vi "kalibrace.vi"() -> ()   [LabVIEW 2024]
uses:
  <vilib>/Analysis/baseanly.llb/Mean (DBL).vi
  EFmeter.lvlib
  <vilib>/Analysis/NI_AALBase.lvlib
  <vilib>/Analysis/NI_AALPro.lvlib
panel:
  out "Polynomial Coefficients":dbl[](array[numeric])
  out "Best Polynomial Fit":dbl[](array[numeric])
  in  "vyh\nVyhodnotit":bool
  in  "Další":bool caption="OK Button"
  in  "Reálná hodnota vstupní veličiny":dbl
  in  "Clear":bool
  in  "Uložit data":bool
  in  "file path (use dialog)":path
  in  "Vzorku na krokù":u16 max=100 step=1
  in  "Prumerovani":bool
  out "error out 2":errorcluster
  in  "VISA resource name 2":refnum<visa-resource-name>
  out "R_out":dbl
  out "XY Graph 2":cluster{"X":dbl[], "Y":dbl[]}[](graph)
  in  "stop":bool
  in  "Start":bool
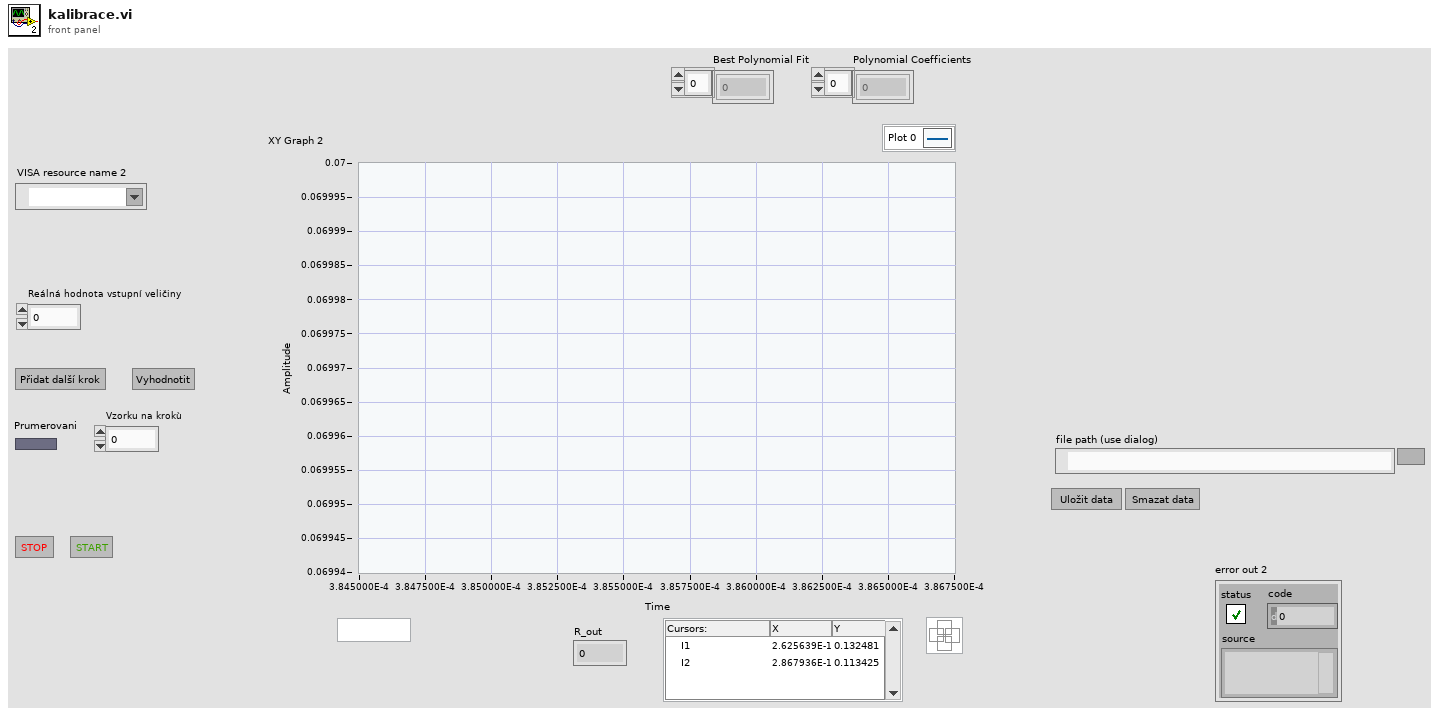
[diagram p1: front panel]
types:
  T1 = enum16{"init", "wait", "graph", "meas", "change_load", "init_measurment", "save", "clear"}
  T2 = typedef "LVCursorListTypeDef.ctl" = cluster{"Name":string, "Color":u32, "Style":u8, "Point Style":u8, "Name Visible":bool, "Allow Drag":bool, "Cursor Mode":u32, "Plot":i32, "Index":i32, "Position":cluster{"X":dbl, "Y":dbl}, "X Scale":u32, "Y Scale":u32, "Watch Plots":i32[], "Watch All Plots":bool, "Plot Area":i32, "Label Offset":cluster{"X":dbl, "Y":dbl}}[]
  T3 = cluster{"Name":string, "Color":u32, "Style":u8, "Point Style":u8, "Name Visible":bool, "Allow Drag":bool, "Cursor Mode":u32, "Plot":i32, "Index":i32, "Position":cluster{"X":dbl, "Y":dbl}, "X Scale":u32, "Y Scale":u32, "Watch Plots":i32[], "Watch All Plots":bool, "Plot Area":i32, "Label Offset":cluster{"X":dbl, "Y":dbl}}
  T4 = enum16{"open", "replace", "create", "open or create", "replace or create", "replace or create with confirmation"}
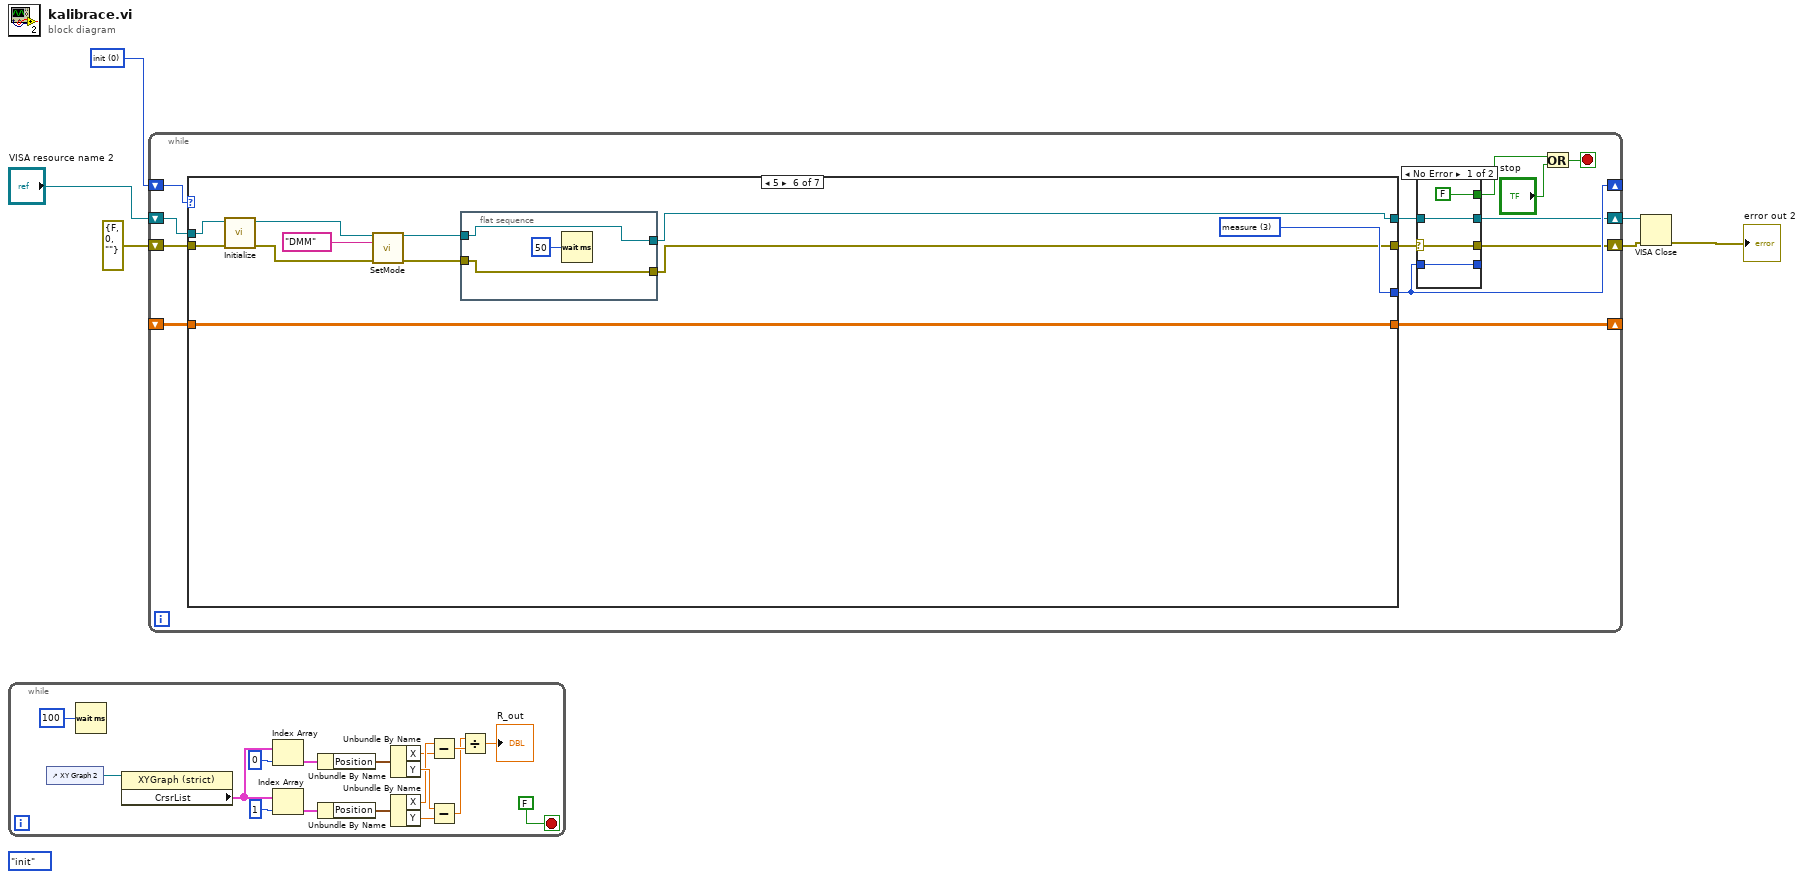
[diagram p0: block diagram]
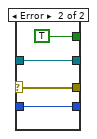
[diagram p2: hidden frame]
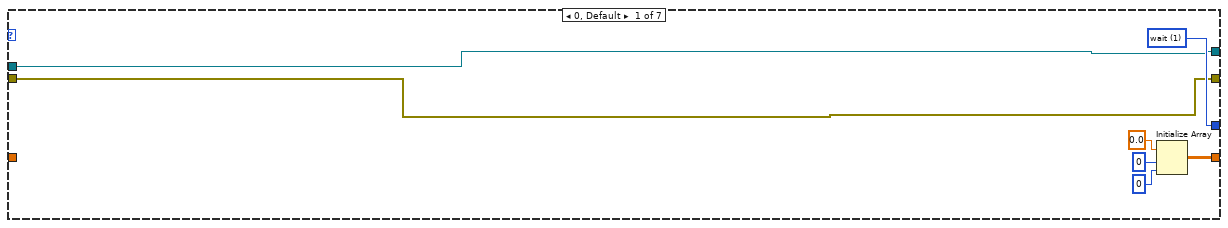
[diagram p3: hidden frame]
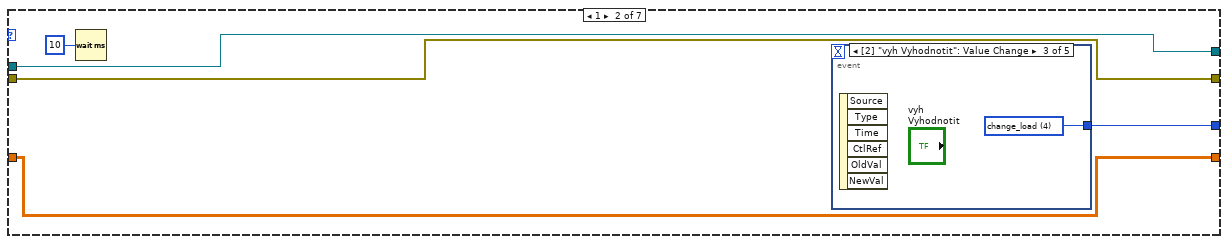
[diagram p4: hidden frame]
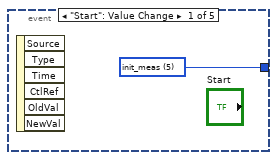
[diagram p5: hidden frame]
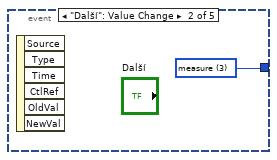
[diagram p6: hidden frame]
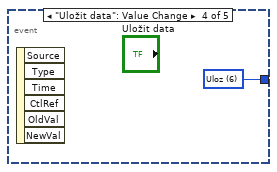
[diagram p7: hidden frame]
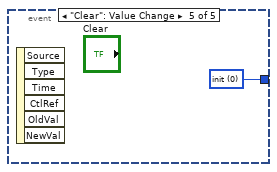
[diagram p8: hidden frame]
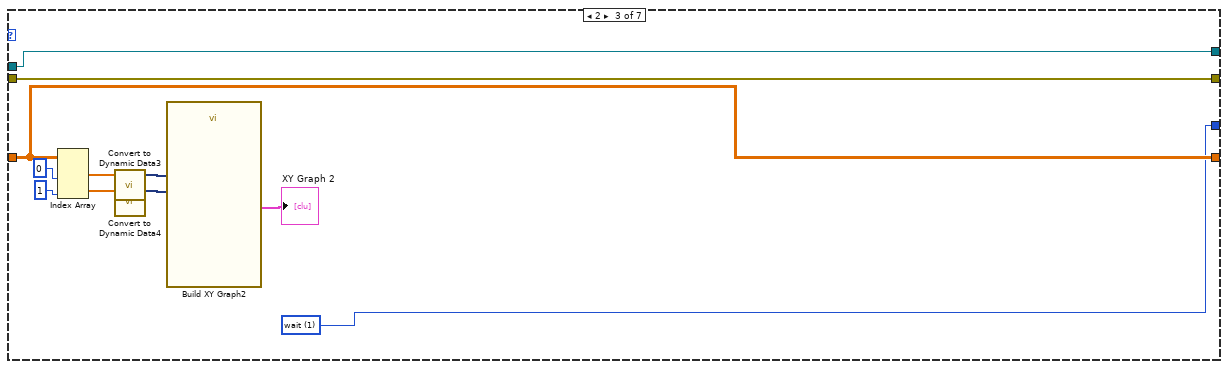
[diagram p9: hidden frame]
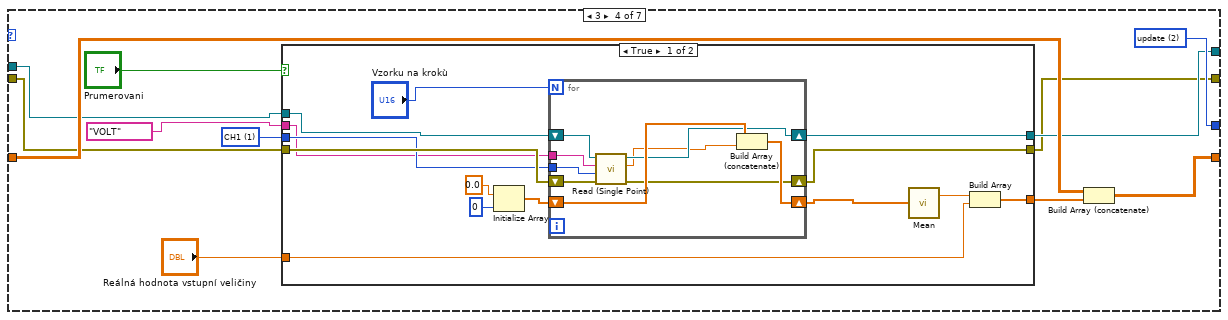
[diagram p10: hidden frame]
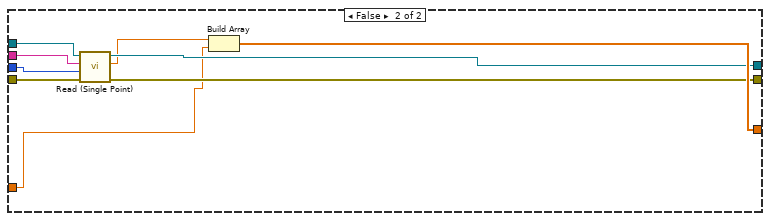
[diagram p11: hidden frame]
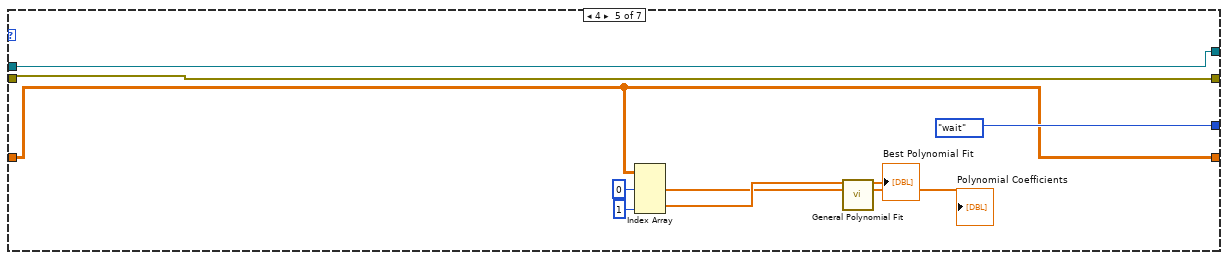
[diagram p12: hidden frame]
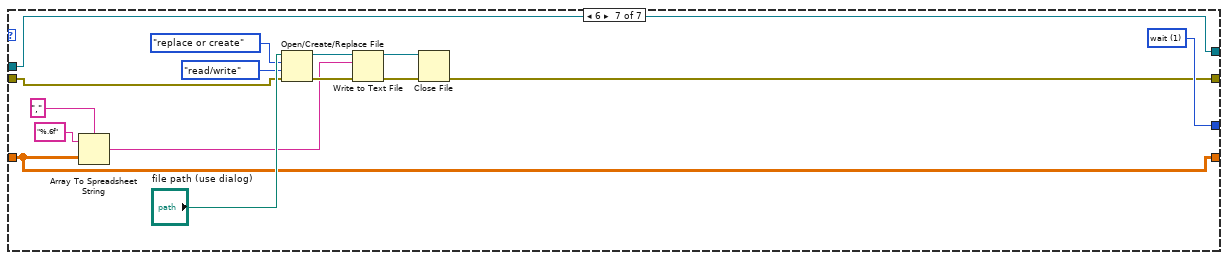
[diagram p13: hidden frame]
diagram:
  (unwired) T1."init"
  w6 = u16 0 items=["init", "wait", "update", "measure", "change_load", "init_meas", "Uloz", "clear"]
  n1 = while {
    stop <- FALSE stop-if-true
    n2 = control-ref of="XY Graph 2"() -> (w21:refnum<vi>)
    n3 = Wait (ms)(milliseconds to wait=u32 100) -> ()  [unwired: 1 out]
    n4 = property class="XYGraph (strict)"(reference=w21) -> ("CrsrList"=w16:T2)  [unwired: 1 in, 2 out]
    n5 = Index Array(array=w16, index=0) -> (element=w22:T3)
    n6 = Index Array(array=w16, index=1) -> (element=w18:T3)
    n7 = Unbundle By Name(w22) -> ("Position"=w23:cluster{"X":dbl, "Y":dbl})
    n8 = Unbundle By Name(w18) -> ("Position"=w19:cluster{"X":dbl, "Y":dbl})
    n9 = Unbundle By Name(w23) -> ("X"=w7:dbl, "Y"=w14:dbl)
    n10 = Unbundle By Name(w19) -> ("X"=w8:dbl, "Y"=w15:dbl)
    n11 = Subtract(x=w8, y=w7) -> (x-y=w10:dbl)
    n12 = Subtract(x=w14, y=w15) -> (x-y=w9:dbl)
    n13 = Divide(x=w9, y=w10) -> (x/y=→"R_out":dbl)
  }
  n14 = while {
    shift-right: [w36] -> _
    shift-left: _ -> [w35]
    shift-right: [w31] -> _
    shift-left: w6 -> [w34]
    shift-right: [w28] -> w2
    shift-left: "VISA resource name 2" -> [w33]
    shift-right: [w27] -> w1
    shift-left: errorcluster {"status"=FALSE, "code"=0, "source"=""} ("error in (no error)") -> [w32]
    stop <- w25 stop-if-true
    n15 = case shown="5" w34 {
      tunnel: [w49 w55 w68 w83 w123 w137 w150] -> w36
      tunnel: w35 -> [_ w55 w68 w84 w123 w137 w150]
      tunnel: [w48 w56 w62 w81 T1."wait" w131 w148] -> w31
      tunnel: [w45 w53 w63 w75 w124 w128 w144] -> w30
      tunnel: [w46 w54 w64 w76 w126 w130 w155] -> w29
      tunnel: w33 -> [w46 w54 w64 w80 w126 w133 w155]
      tunnel: w32 -> [w45 w53 w63 w79 w124 w132 w151]
      frame 0, Default {
        w48 = u16 1 items=["init", "wait", "update", "measure"]
        n16 = Initialize Array(0.0 ("element"), 0 ("dimension size"), 0 ("dimension size")) -> (w49:dbl[][])
      }
      frame 1 {
        n17 = Wait (ms)(milliseconds to wait=u32 10) -> ()  [unwired: 1 out]
        n18 = event shown="[2] \"vyh Vyhodnotit\": Value Change" {
          selector: _ -> [_ _ _ _ _]
          dyn-events: _ -> [_ _ _ _ _]
          timeout: _ -> [_ _ _ _ _]
          tunnel: [w57 w58 w59 w60 w61] -> w56
          event "Start": Value Change {
            w57 = u16 5 items=["init", "wait", "update", "measure", "change_load", "init_meas"]
            n19 = event-data() -> ()  [unwired: 1 in, 6 out]
          }
          event "Další": Value Change {
            w58 = u16 3 items=["init", "wait", "update", "measure", "change_load", "init_meas", "Uloz", "clear"]
            n20 = event-data() -> ()  [unwired: 1 in, 6 out]
          }
          event "vyh\nVyhodnotit": Value Change {
            w59 = u16 4 items=["init", "wait", "update", "measure", "change_load", "init_meas", "Uloz", "clear"]
            n21 = event-data() -> ()  [unwired: 1 in, 6 out]
          }
          event "Uložit data": Value Change {
            w60 = u16 6 items=["init", "wait", "update", "measure", "change_load", "init_meas", "Uloz"]
            n22 = event-data() -> ()  [unwired: 1 in, 6 out]
          }
          event "Clear": Value Change {
            w61 = u16 0 items=["init", "wait", "update", "measure", "change_load", "init_meas", "Uloz", "clear"]
            n23 = event-data() -> ()  [unwired: 1 in, 6 out]
          }
        }
      }
      frame 2 {
        w62 = u16 1 items=["init", "wait", "update", "measure"]
        n24 = Index Array(array=w68, index (col) #1=0 ("index (row)"), index (col) #2=1 ("index (row)")) -> (element #1=w72:dbl[], element #2=w69:dbl[])  [unwired: 2 in]
        n25 = call "Convert to Dynamic Data3"("Array"=w72) -> ("Dynamic Data Type"=w71:dynamicdata)  [unwired: 3 in]
        n26 = call "Convert to Dynamic Data4"("Array"=w69) -> ("Dynamic Data Type"=w70:dynamicdata)  [unwired: 3 in]
        n27 = call "Build XY Graph2"("Y Input"=w70, "X Input"=w71) -> ("XY Graph"=→"XY Graph 2":cluster{"X":dbl[], "Y":dbl[]}[])  [unwired: 8 in, 1 out]
      }
      frame 3 {
        w78 = u16 1 items=["CH2"=2, "CH1"=1] ("Ring")
        w81 = u16 2 items=["init", "wait", "update", "measure"]
        n28 = case shown="True" "Prumerovani" {
          tunnel: [w89 w116] -> w82
          tunnel: w80 -> [w94 w115]
          tunnel: w79 -> [w93 w114]
          tunnel: w78 -> [w92 w113]
          tunnel: "VOLT" ("Combo Box") -> [w91 w112]
          tunnel: [w88 w110] -> w76
          tunnel: [w87 w111] -> w75
          tunnel: "Reálná hodnota vstupní veličiny" -> [w85 w109]
          frame True {
            n29 = Initialize Array(0.0 ("element"), 0 ("dimension size")) -> (w95:dbl[])
            n30 = for {
              N: "Vzorku na krokù" -> [_]
              shift-right: [w101] -> w88
              shift-left: w94 -> [w106]
              shift-right: [w99] -> w87
              shift-left: w93 -> [w105]
              tunnel: w92 -> [w104]
              tunnel: w91 -> [w103]
              shift-right: [w102] -> w86
              shift-left: w95 -> [w107]
              n31 = call "Read (Single Point).vi"("error in (no error)"=w105, "Ring"=w104, "Combo Box"=w103, "VISA resource name"=w106) -> ("error out"=w99:errorcluster, "Measurement"=w100:dbl, "VISA resource name out"=w101:refnum<visa-resource-name>)  [unwired: 5 in]
              n32 = Build Array (concatenate)(w107, w100) -> (w102:dbl[])
            }
            n33 = call-poly <vilib>:"Mean.vi"("X"=w86) -> ("mean"=w90:dbl)  [unwired: 1 out]
            n34 = Build Array(w90, w85) -> (w89:dbl[])
          }
          frame False {
            n35 = call "Read (Single Point).vi"("error in (no error)"=w114, "Ring"=w113, "Combo Box"=w112, "VISA resource name"=w115) -> ("error out"=w111:errorcluster, "Measurement"=w108:dbl, "VISA resource name out"=w110:refnum<visa-resource-name>)  [unwired: 5 in]
            n36 = Build Array(w108, w109) -> (w116:dbl[])
          }
        }
        n37 = Build Array (concatenate)(w84, w82) -> (w83:dbl[][])
      }
      frame 4 {
        n38 = Index Array(array=w123, index (col) #1=0 ("disabled index (col)"), index (col) #2=1 ("disabled index (col)")) -> (element #1=w119:dbl[], element #2=w120:dbl[])  [unwired: 2 in]
        n39 = call <vilib>:"General Polynomial Fit.vi"("Y"=w120, "X"=w119) -> ("Best Polynomial Fit"=→"Best Polynomial Fit":dbl[], "Polynomial Coefficients"=→"Polynomial Coefficients":dbl[])  [unwired: 10 in, 2 out]
      }
      frame 5 {
        w131 = u16 3 items=["init", "wait", "update", "measure", "change_load", "init_meas"]
        n40 = call "Initialize.vi"("error in (no error)"=w132, "VISA resource name"=w133) -> ("error out"=w136:errorcluster, "VISA resource name out"=w135:refnum<visa-resource-name>)  [unwired: 8 in]
        n41 = call "SetMode.vi"("VISA resource name"=w135, "Combo Box"="DMM", "error in (no error)"=w136) -> ("VISA resource name out"=w129:refnum<visa-resource-name>, "error out"=w127:errorcluster)  [unwired: 11 in]
        n42 = flat-sequence {
          tunnel: [w139] -> w130
          tunnel: w129 -> [w139]
          tunnel: w127 -> [w138]
          tunnel: [w138] -> w128
          frame #0 {
            n43 = Wait (ms)(milliseconds to wait=u32 50) -> ()  [unwired: 1 out]
          }
        }
      }
      frame 6 {
        w148 = u16 1 items=["init", "wait", "update", "measure", "change_load", "init_meas"]
        n44 = Array To Spreadsheet String(delimiter (Tab)=",", array=w150, 3:"%.6f" ("format string")) -> (spreadsheet string=w141:string)
        n45 = Open/Create/Replace File(file path (use dialog)="file path (use dialog)", error in=w151, operation (0:open)=T4."replace or create", access (0:read/write)=enum16{"read/write", "read-only", "write-only"}."read/write") -> (refnum out=w143:refnum<file>, error out=w146:errorcluster)  [unwired: 2 in, 1 out]
        n46 = Write to Text File(file (use dialog)=w143, text=w141, error in=w146) -> (refnum out=w142:refnum<file>, error out=w145:errorcluster)  [unwired: 1 in, 1 out]
        n47 = Close File(refnum=w142, error in=w145) -> (error out=w144:errorcluster)  [unwired: 1 out]
      }
    }
    n48 = case shown="No Error" w30 {
      selector: w30 -> [w38 w42]
      tunnel: w31 -> [w40 w43]
      tunnel: [w40 w43] -> _
      tunnel: w29 -> [w39 w44]
      tunnel: [w39 w44] -> w28
      tunnel: [w38 w42] -> w27
      tunnel: [FALSE TRUE] -> w24
      frame No Error {
      }
      frame Error {
      }
    }
    n49 = Or(x=w24, y="stop") -> (x .or. y?=w25:bool)
  }
  n50 = VISA Close(VISA resource name=w2, error in (no error)=w1) -> (error out=→"error out 2":errorcluster)
